vi "Generate license file for that machine.vi"(8 "error in (no error)":errorcluster, 9 "MAC address":string, 10 "prefix text":string="tctechinc", 11 "folder path":path) -> (0 "error out":errorcluster, 3 "file path":path)   [LabVIEW 2016]
doc: "Generate license file with the information of a MAC address and the <b>prefix text</b>. The <b>folder path</b> is assigned as the container of the license file in the <b>file path</b>. If the <b>folder path</b> is empty, the license file is generated and located in the same folder as this VI."
panel:
  out "MD5 Message Digest":string
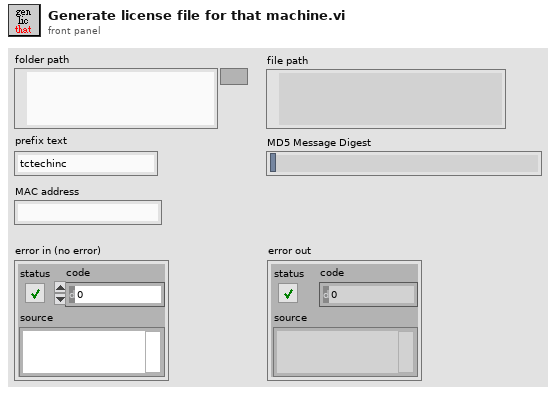
[diagram p1: front panel]
types:
  T1 = enum16{"open", "replace", "create", "open or create", "replace or create", "replace or create with confirmation"}
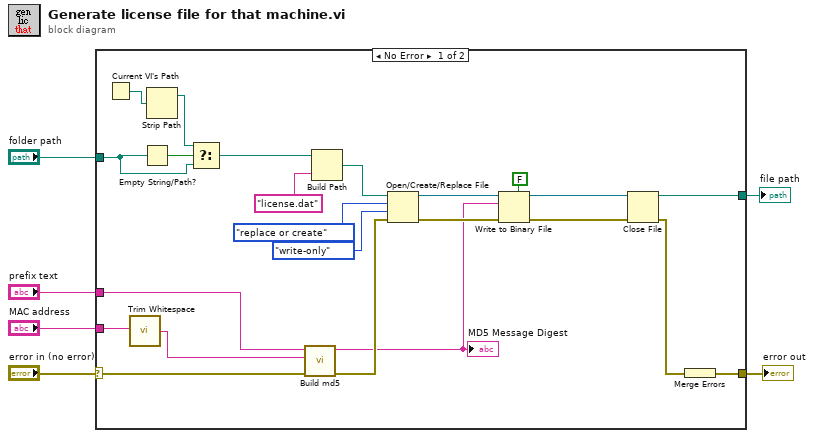
[diagram p0: block diagram]
diagram:
  n1 = case shown="No Error" "error in (no error)" {
    selector: "error in (no error)" -> [w11 w30]
    tunnel: [w21 _] -> w6
    tunnel: [w19 w30] -> w4
    tunnel: "prefix text" -> [w12 _]
    tunnel: "folder path" -> [w14 _]
    tunnel: "MAC address" -> [w8 _]
    frame No Error {
      n2 = Current VI's Path() -> (path=w17:path)
      n3 = call <vilib>:"Trim Whitespace.vi"("string"=w8) -> ("trimmed string"=w7:string)  [unwired: 1 in]
      n4 = Empty String/Path?(string/path=w14) -> (empty?=w16:bool)
      n5 = Strip Path(path=w17) -> (stripped path=w15:path)  [unwired: 1 out]
      n6 = Select(t=w15, s=w16, f=w14) -> (s? t:f=w13:path)
      n7 = call "Build md5.vi"("error in (no error)"=w11, "words"=w7, "prefix"=w12) -> ("error out"=w10:errorcluster, "MD5 Message Digest"=w9:string)  [unwired: 7 in]
      "MD5 Message Digest" <- w9
      n8 = Build Path(base path=w13, name or relative path="license.dat") -> (appended path=w24:path)
      n9 = Open/Create/Replace File(file path (use dialog)=w24, error in=w10, operation (0:open)=T1."replace or create", access (0:read/write)=enum16{"read/write", "read-only", "write-only"}."write-only") -> (refnum out=w28:refnum<file>, error out=w27:errorcluster)  [unwired: 2 in, 1 out]
      n10 = Write to Binary File(file (use dialog)=w28, data=w9, error in=w27, 5:FALSE ("prepend array or string size? (T)")) -> (refnum out=w26:refnum<file>, error out=w25:errorcluster)  [unwired: 2 in, 1 out]
      n11 = Close File(refnum=w26, error in=w25) -> (path=w21:path, error out=w20:errorcluster)
      n12 = Merge Errors(w20) -> (w19:errorcluster)
    }
    frame Error {
    }
  }
  "error out" <- w4
  "file path" <- w6
